vi "BackgroundTests.vi"() -> ()   [LabVIEW 2023]
panel:
  in  "stop":bool
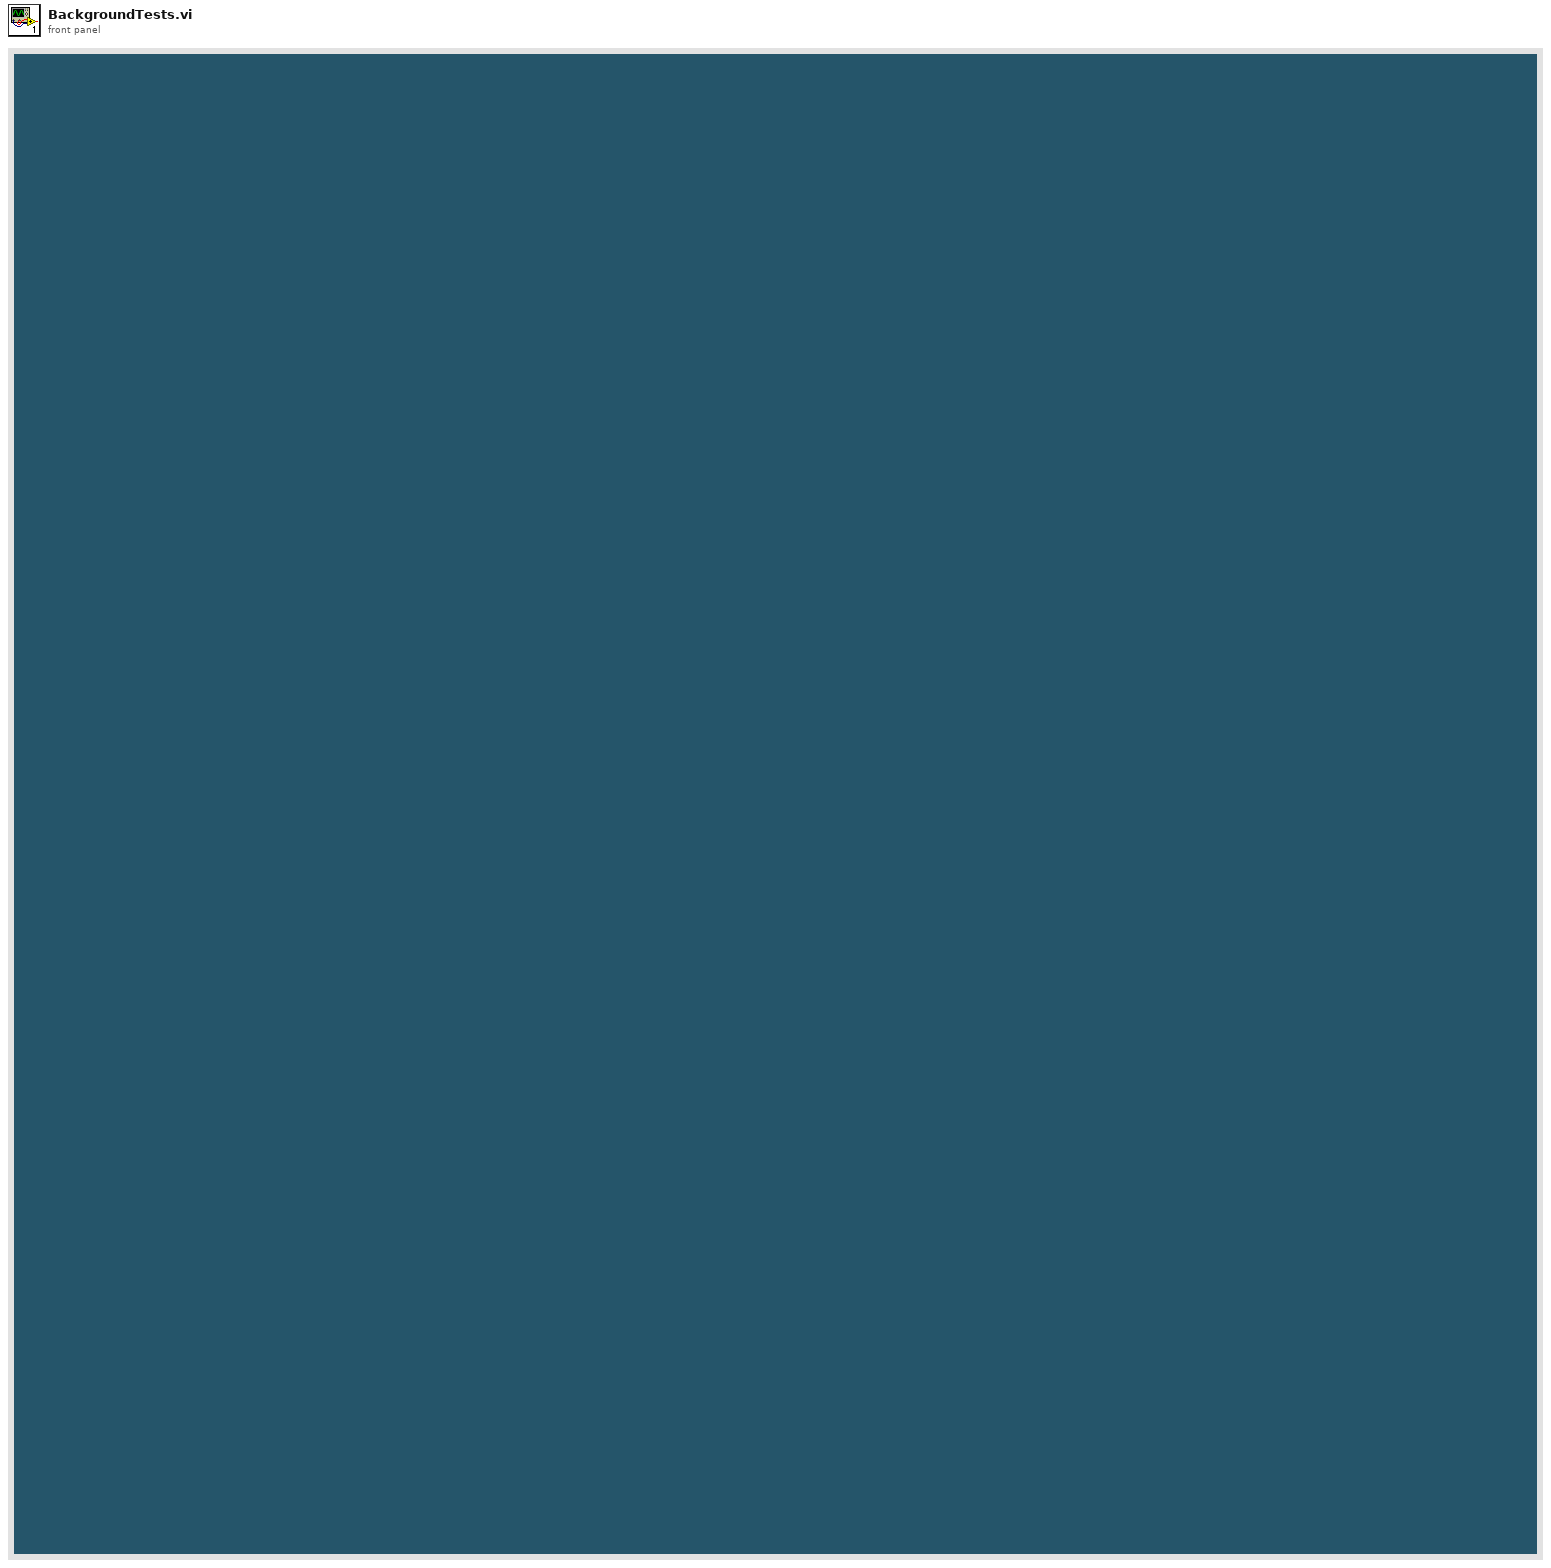
[diagram p1: front panel]
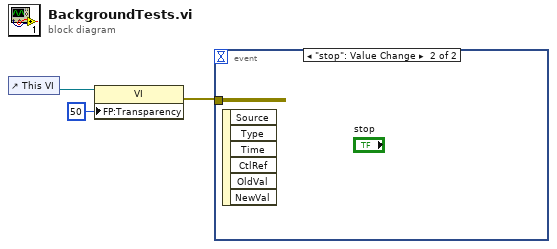
[diagram p0: block diagram]
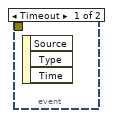
[diagram p2: hidden frame]
diagram:
  n1 = control-ref of="This VI"() -> (w2:refnum<vi>)
  n2 = property class="VI"(reference=w2, "FP:Transparency"=u8 50 ("Front Panel Window:Transparency")) -> (error out=w1:errorcluster)  [unwired: 1 in, 1 out]
  n3 = event shown="[1] \"stop\": Value Change" {
    selector: _ -> [_ _]
    dyn-events: _ -> [_ _]
    timeout: _ -> [_ _]
    tunnel: w1 -> [_ _]
    event Timeout {
      n4 = event-data() -> ()  [unwired: 1 in, 3 out]
    }
    event "stop": Value Change {
      n5 = event-data() -> ()  [unwired: 1 in, 6 out]
    }
  }
